vi "mxwScript_Cmnd2Str_addCleanupOption.vi"(8 "error in (no error)":errorcluster, 11 "data":variant) -> (0 "error out":errorcluster, 3 "outputString":string)   [LabVIEW 2020]
uses:
  codeGenAPISupport.llb/cgAPI_mxwScript_Cleanup_Option.ctl
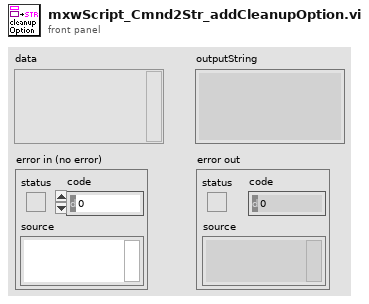
[diagram p1: front panel]
types:
  T1 = typedef "cgAPI_mxwScript_Cleanup_Option.ctl" = cluster{"name":string, "data":string, "location":i32}
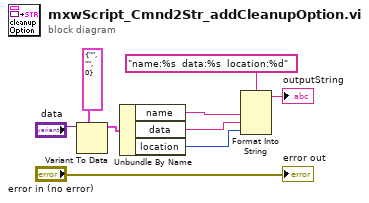
[diagram p0: block diagram]
diagram:
  n1 = Variant To Data(type=T1 {"name"="", "data"="", "location"=0} ("cleanupOption"), Variant="data") -> (data=w8:T1)  [unwired: 1 in, 1 out]
  n2 = Unbundle By Name(w8) -> ("name"=w5:string, "data"=w4:string, "location"=w3:i32)
  n3 = Format Into String(format string="name:%s  data:%s  location:%d", w5, w4, w3) -> (resulting string=→"outputString":string)  [unwired: 2 in, 1 out]
  "error out" <- "error in (no error)"
